vi "find average of coordinates.vi"() -> ()   [LabVIEW 2021]
uses:
  <vilib>/Utility/file.llb/Write Delimited Spreadsheet (DBL).vi
panel:
  out "x/y":dbl[](array[numeric]) format="%.6g"
  out "transposed array":dbl[][](array[numeric]) format="%.6g"
  out "array":dbl[][](array[numeric]) format="%.6g"
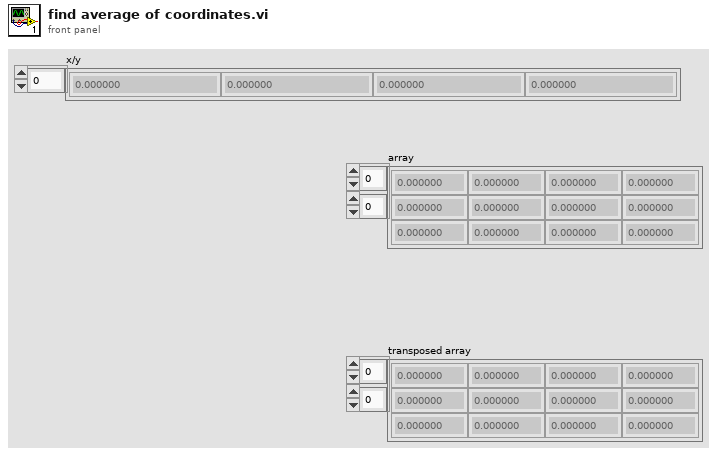
[diagram p1: front panel]
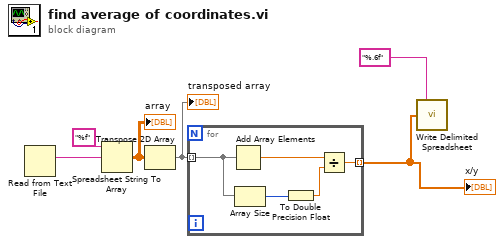
[diagram p0: block diagram]
diagram:
  n1 = Read from Text File() -> (text=w6:string)  [unwired: 4 in, 3 out]
  n2 = Spreadsheet String To Array(format string="%f", spreadsheet string=w6) -> (array=w4:dbl[][])  [unwired: 2 in]
  "array" <- w4
  n3 = Transpose 2D Array(2D array=w4) -> (transposed array=w3:dbl[][])
  "transposed array" <- w3
  n4 = for {
    tunnel: w3 -> [w10] mode=indexing
    tunnel: [w7] -> w2 mode=indexing
    n5 = Add Array Elements(numeric array=w10) -> (sum=w8:dbl)
    n6 = Array Size(array=w10) -> (size(s)=w9:i32)
    n7 = To Double Precision Float(number=w9) -> (double precision float=w11:dbl)
    n8 = Divide(x=w8, y=w11) -> (x/y=w7:dbl)
  }
  "x/y" <- w2
  n9 = call-poly <vilib>:"Write Delimited Spreadsheet.vi"("format (%.3f)"="%.6f", "1D data"=w2) -> ()  [unwired: 12 in, 2 out]
